vi "Camera Settings to INI Section.vi"(6 "do not save":string[](array[string]), 8 "error in (no error)":errorcluster, 9 "Filters":string[](array[string]), 10 "refnum in":T1, 11 "IMAQdx Cam in":refnum<class "IMAQdx Cam.lvclass">) -> (0 "error out":errorcluster, 2 "refnum out":T1, 3 "IMAQdx Cam out":refnum<class "IMAQdx Cam.lvclass">)   [LabVIEW 2020, in "IMAQdx Cam.lvclass"]
uses:
  IMAQdx Cam.lvclass
  <vilib>/Utility/config.llb/Config Data RefNum.ctl
  IMAQdx Cam.lvclass/IMAQdx Cam.ctl
  <vilib>/Utility/config.llb/Write Key (String).vi
  <vilib>/Utility/config.llb/Write Key (U32).vi
  <vilib>/Utility/config.llb/Write Key (Double).vi
  <vilib>/Utility/config.llb/Write Key (Boolean).vi
  <vilib>/vision/driver/NI_Vision_Acquisition_Software.lvlib
  <resource>/objmgr/imaqdx.rc
  <vilib>/Utility/config.llb/NI_LVConfig.lvlib
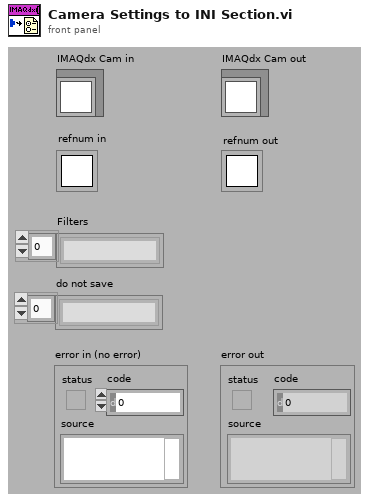
[diagram p1: front panel]
types:
  T1 = typedef "NI_LVConfig.lvlib/Config Data RefNum.ctl" = refnum<k1>
  T2 = enum16{"fractional", "engineering", "exponential"}
  T3 = typedef "IMAQdx.ctl" = refnum<k21>
  T4 = typedef "NI_Vision_Acquisition_Software.lvlib/IMAQdx Attribute Type.ctl" = enum32{"U32", "I64", "DBL", "String", "Enum", "Bool", "Command"}
  T5 = cluster{"Attribute Type":T4, "Readable":bool, "Writable":bool, "Attribute Name":string}[]
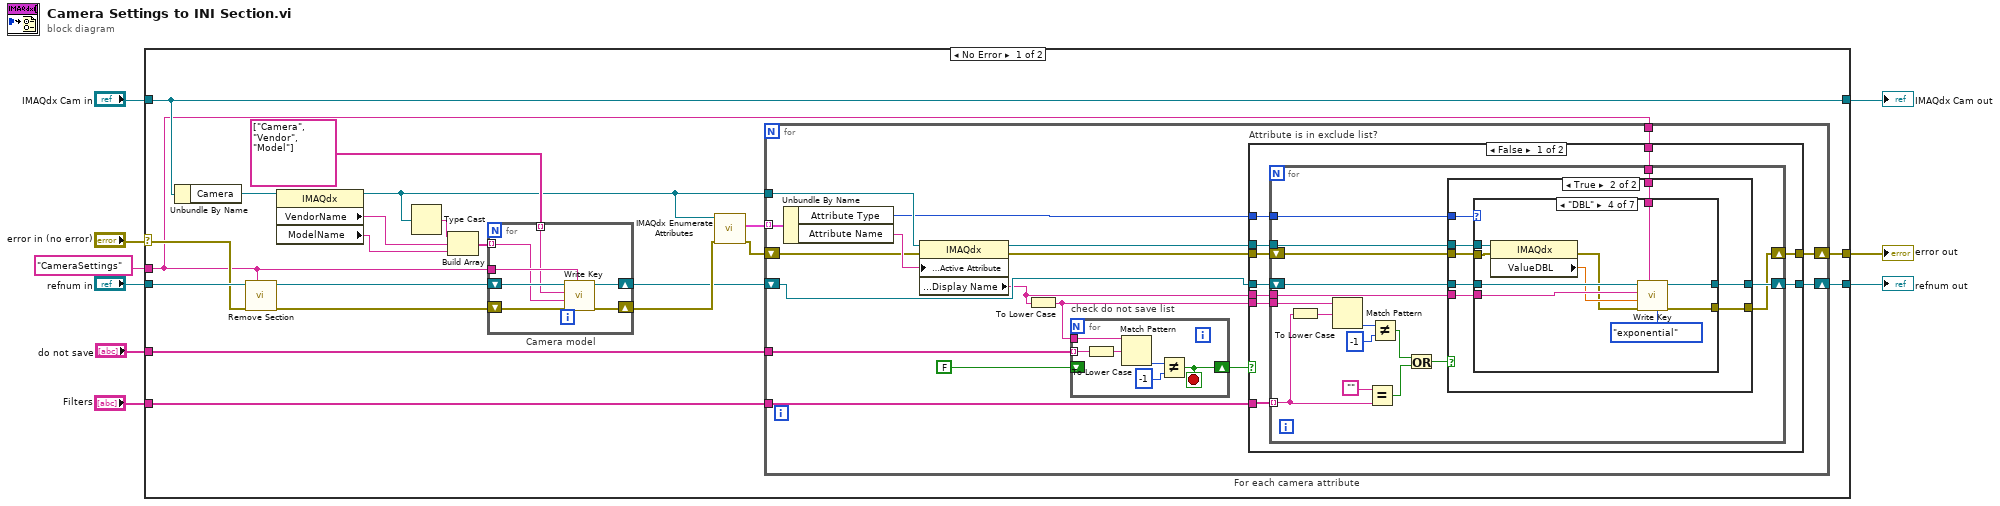
[diagram p0: block diagram]
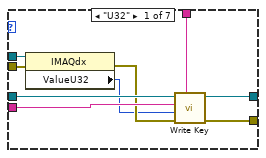
[diagram p3: hidden frame]
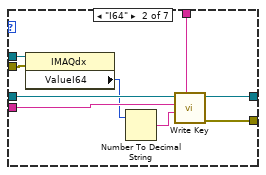
[diagram p4: hidden frame]
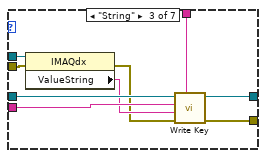
[diagram p5: hidden frame]
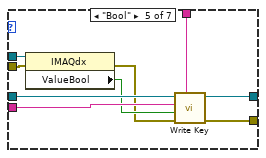
[diagram p6: hidden frame]
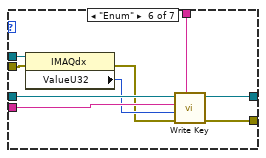
[diagram p7: hidden frame]
diagram:
  n1 = case shown="No Error" "error in (no error)" {
    selector: "error in (no error)" -> [w22 w159]
    tunnel: [w25 w159] -> w8
    tunnel: [w27 w158] -> w6
    tunnel: "IMAQdx Cam in" -> [w27 w158]
    tunnel: "Filters" -> [w30 _]
    tunnel: "CameraSettings" -> [w16 _]
    tunnel: "refnum in" -> [w23 w157]
    tunnel: [w28 w157] -> w2
    tunnel: "do not save" -> [w24 _]
    frame No Error {
      n2 = Unbundle By Name(w27) -> ("Camera"=w12:T3)
      n3 = call <vilib>:"Remove Section.vi"("section"=w16, "error in (no error)"=w22, "refnum"=w23) -> ("error out"=w17:errorcluster, "refnum out"=w18:T1)  [unwired: 6 in, 1 out]
      n4 = property class="IMAQdx"(reference=w12) -> (reference out=w11:T3, "VendorName"=w21:string, "ModelName"=w20:string)  [unwired: 1 in, 1 out]
      n5 = Type Cast(x=w11) -> (*(type *) &x=w19:string)  [unwired: 1 in]
      n6 = Build Array(w19, w21, w20) -> (w15:string[])
      n7 = for "Camera model" {
        shift-right: [w32] -> w14
        shift-left: w17 -> [w36]
        shift-right: [w34] -> w10
        shift-left: w18 -> [w37]
        tunnel: w16 -> [w35]
        tunnel: w15 -> [w33] mode=indexing
        tunnel: string[] ["Camera", "Vendor", "Model"] -> [w31] mode=indexing
        n8 = call-poly <vilib>:"Write Key.vi"("section"=w35, "error in (no error)"=w36, "value"=w33, "key"=w31, "refnum"=w37) -> ("error out"=w32:errorcluster, "refnum out"=w34:T1)  [unwired: 4 in, 1 out]
      }
      n9 = call <vilib>:"IMAQdx Enumerate Attributes.vi"("error in"=w14, "Session In"=w11) -> ("error out"=w26:errorcluster, "Attribute Information Array"=w29:T5)  [unwired: 7 in, 1 out]
      n10 = for "For each camera attribute" {
        tunnel: w30 -> [w53]
        tunnel: w29 -> [w54] mode=indexing
        tunnel: w11 -> [w52]
        tunnel: w16 -> [w49]
        shift-right: [w47] -> w28
        shift-left: w10 -> [w48]
        shift-right: [w44] -> w25
        shift-left: w26 -> [w43]
        tunnel: w24 -> [w41]
        n11 = Unbundle By Name(w54) -> ("Attribute Type"=w50:T4, "Attribute Name"=w51:string)
        n12 = property class="IMAQdx"(reference=w52, error in=w43, "Camera Attributes:Active Attribute"=w51) -> (reference out=w45:T3, error out=w46:errorcluster, "Camera Attributes:Display Name"=w42:string)
        n13 = To Lower Case(string=w42) -> (all lower case string=w38:string)
        n14 = for "check do not save list" {
          tunnel: w41 -> [w156] mode=indexing
          shift-right: [w153] -> w39
          shift-left: FALSE -> [_]
          tunnel: w38 -> [w151]
          stop <- w153 stop-if-true
          n15 = To Lower Case(string=w156) -> (all lower case string=w152:string)
          n16 = Match Pattern(string=w151, regular expression=w152) -> (offset past match=w155:i32)  [unwired: 1 in, 3 out]
          n17 = Not Equal?(x=w155, y=-1) -> (x != y?=w153:bool)
        }
        n18 = case "Attribute is in exclude list?" shown="False" w39 {
          tunnel: w53 -> [w64 _]
          tunnel: w50 -> [w63 _]
          tunnel: w49 -> [w62 _]
          tunnel: w48 -> [w61 w150]
          tunnel: [w60 w150] -> w47
          tunnel: w46 -> [w59 w149]
          tunnel: w45 -> [w58 _]
          tunnel: [w57 w149] -> w44
          tunnel: w42 -> [w56 _]
          tunnel: w38 -> [w55 _]
          frame False {
            n19 = for {
              tunnel: w64 -> [w73] mode=indexing
              tunnel: w56 -> [w74]
              tunnel: w63 -> [w75]
              tunnel: w62 -> [w72]
              shift-right: [w70] -> w60
              shift-left: w61 -> [w71]
              tunnel: w58 -> [w69]
              shift-right: [w67] -> w57
              shift-left: w59 -> [w68]
              tunnel: w55 -> [w65]
              n20 = To Lower Case(string=w73) -> (all lower case string=w81:string)
              n21 = Match Pattern(string=w65, regular expression=w81) -> (offset past match=w77:i32)  [unwired: 1 in, 3 out]
              n22 = Equal?(x="", y=w73) -> (x = y?=w79:bool)
              n23 = Not Equal?(x=w77, y=-1) -> (x != y?=w80:bool)
              n24 = Or(x=w80, y=w79) -> (x .or. y?=w66:bool)
              n25 = case shown="True" w66 {
                tunnel: w75 -> [_ w91]
                tunnel: w74 -> [_ w90]
                tunnel: w72 -> [_ w89]
                tunnel: w71 -> [w83 w88]
                tunnel: [w83 w87] -> w70
                tunnel: w69 -> [_ w86]
                tunnel: w68 -> [w82 w85]
                tunnel: [w82 w84] -> w67
                frame False {
                }
                frame True {
                  n26 = case shown="\"DBL\"" w91 {
                    tunnel: w90 -> [w98 w109 w118 w128 w137 w146 _]
                    tunnel: w89 -> [w96 w108 w117 w127 w136 w145 _]
                    tunnel: w88 -> [w97 w107 w116 w126 w135 w144 w148]
                    tunnel: [w95 w106 w115 w125 w134 w143 w148] -> w87
                    tunnel: w86 -> [w100 w105 w114 w124 w133 w142 _]
                    tunnel: w85 -> [w99 w104 w113 w123 w132 w141 w147]
                    tunnel: [w93 w101 w110 w120 w130 w139 w147] -> w84
                    frame "U32" {
                      n27 = property class="IMAQdx"(reference=w100, error in=w99) -> (error out=w94:errorcluster, "ValueU32"=w92:u32)  [unwired: 1 out]
                      n28 = call-poly <vilib>:"Write Key.vi"("section"=w96, "error in (no error)"=w94, "value"=w92, "key"=w98, "refnum"=w97) -> ("error out"=w93:errorcluster, "refnum out"=w95:T1)  [unwired: 4 in, 1 out]
                    }
                    frame "I64" {
                      n29 = property class="IMAQdx"(reference=w105, error in=w104) -> ("ValueI64"=w103:i64)  [unwired: 2 out]
                      n30 = Number To Decimal String(number=w103) -> (decimal integer string=w102:string)  [unwired: 1 in]
                      n31 = call-poly <vilib>:"Write Key.vi"("section"=w108, "value"=w102, "key"=w109, "refnum"=w107) -> ("error out"=w101:errorcluster, "refnum out"=w106:T1)  [unwired: 5 in, 1 out]
                    }
                    frame "String" {
                      n32 = property class="IMAQdx"(reference=w114, error in=w113) -> (error out=w111:errorcluster, "ValueString"=w112:string)  [unwired: 1 out]
                      n33 = call-poly <vilib>:"Write Key.vi"("section"=w117, "error in (no error)"=w111, "value"=w112, "key"=w118, "refnum"=w116) -> ("error out"=w110:errorcluster, "refnum out"=w115:T1)  [unwired: 4 in, 1 out]
                    }
                    frame "DBL" {
                      n34 = property class="IMAQdx"(reference=w124, error in=w123) -> (error out=w119:errorcluster, "ValueDBL"=w122:dbl)  [unwired: 1 out]
                      n35 = call-poly <vilib>:"Write Key.vi"("format (fractional)"=T2."exponential", "section"=w127, "error in (no error)"=w119, "value"=w122, "key"=w128, "refnum"=w126) -> ("error out"=w120:errorcluster, "refnum out"=w125:T1)  [unwired: 3 in, 1 out]
                    }
                    frame "Bool" {
                      n36 = property class="IMAQdx"(reference=w133, error in=w132) -> (error out=w129:errorcluster, "ValueBool"=w131:bool)  [unwired: 1 out]
                      n37 = call-poly <vilib>:"Write Key.vi"("section"=w136, "error in (no error)"=w129, "value"=w131, "key"=w137, "refnum"=w135) -> ("error out"=w130:errorcluster, "refnum out"=w134:T1)  [unwired: 4 in, 1 out]
                    }
                    frame "Enum" {
                      n38 = property class="IMAQdx"(reference=w142, error in=w141) -> (error out=w138:errorcluster, "ValueU32"=w140:u32)  [unwired: 1 out]
                      n39 = call-poly <vilib>:"Write Key.vi"("section"=w145, "error in (no error)"=w138, "value"=w140, "key"=w146, "refnum"=w144) -> ("error out"=w139:errorcluster, "refnum out"=w143:T1)  [unwired: 4 in, 1 out]
                    }
                    frame "Command", Default {
                    }
                  }
                }
              }
            }
          }
          frame True {
          }
        }
      }
    }
    frame Error {
    }
  }
  "error out" <- w8
  "IMAQdx Cam out" <- w6
  "refnum out" <- w2
